vi "Encoder Follower.vi"() -> ()   [LabVIEW 2018]
panel:
  in  "Encoder Configuration":T1
  in  "PIDVA":T2
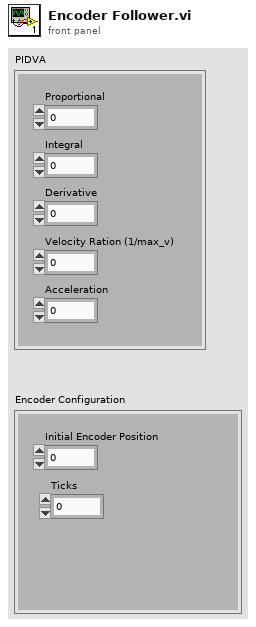
[diagram p1: front panel]
types:
  T1 = cluster{"Initial Encoder Position":dbl, "Ticks":dbl}
  T2 = cluster{"Proportional":dbl, "Integral":dbl, "Derivative":dbl, "Velocity Ration (1/max_v)":dbl, "Acceleration":dbl}
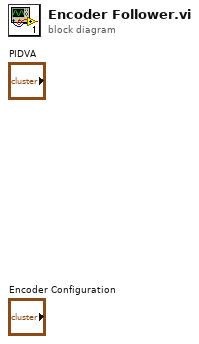
[diagram p0: block diagram]
diagram:
